vi "add_time.vi"   [LabVIEW 2013]
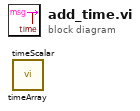
[diagram p0: block diagram]
diagram:
  n1 = call "timeArray.vi"() -> ()  [unwired: 5 in, 1 out]
  n2 = call "timeScalar.vi"() -> ()  [unwired: 5 in, 1 out]
